vi "Manipulator Intake Handler.vi"(0 "Driver Axes":dbl[](array[numeric]), 1 "Driver Buttons":bool[](array[boolean]), 2 "Driver POVs":i16[](array[numeric]), 3 "Operator Axes":dbl[](array[numeric]), 4 "Operator Buttons":bool[](array[boolean]), 5 "Operator POVs":i16[](array[numeric])) -> ()   [LabVIEW 2020]
uses:
  <vilib>/Rock Robotics/WPI/Joystick/XBox Axes Indexer.ctl
  <vilib>/Rock Robotics/WPI/Joystick/XBox Buttons Indexer.ctl
  74f8955f-b1fa-4a71-b90e-be9672dc2c54.vi
  ec023221-8c5a-475e-8a5e-13ba12a89865.vi
  manipulator/Implementation/Typedefs/game object.ctl
  manipulator/Implementation/Typedefs/Cascade Height.ctl
  manipulator/Implementation/manipulator Operations.ctl
  manipulator/Implementation/Typedefs/Teleop Manipulator Commands.ctl
  52cbdbc3-376d-4ae6-b30b-ce1f15df8f80.vi
  dadffdc7-6345-417f-8810-915f08729db8.vi
  b64dc491-ae41-4b64-be03-725d494c7d40.vi
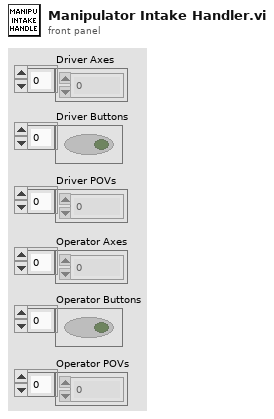
[diagram p1: front panel]
types:
  T1 = typedef "XBox Buttons Indexer.ctl" = enum16{"A", "B", "X", "Y", "Left Bumper", "Right Bumper", "Back", "Start", "Left Joystick", "Right Joystick"}
  T2 = typedef "Teleop Manipulator Commands.ctl" = enum16{"idle", "intake cone", "intake cube", "score low cone", "score low cube", "score mid cone", "score mid cube", "score high cone", "score high cube"}
  T3 = typedef "manipulator Operations.ctl" = enum16{"Reserve", "Read Current", "Immediate", "Reset Manipulator", "Grid-dy"}
  T4 = typedef "XBox Axes Indexer.ctl" = enum16{"Left X", "Left Y", "Left Trigger", "Right Trigger", "Right X", "Right Y"}
  T5 = typedef "game object.ctl" = enum16{"cone", "cube"}
  T6 = typedef "Cascade Height.ctl" = enum16{"Middle", "High"}
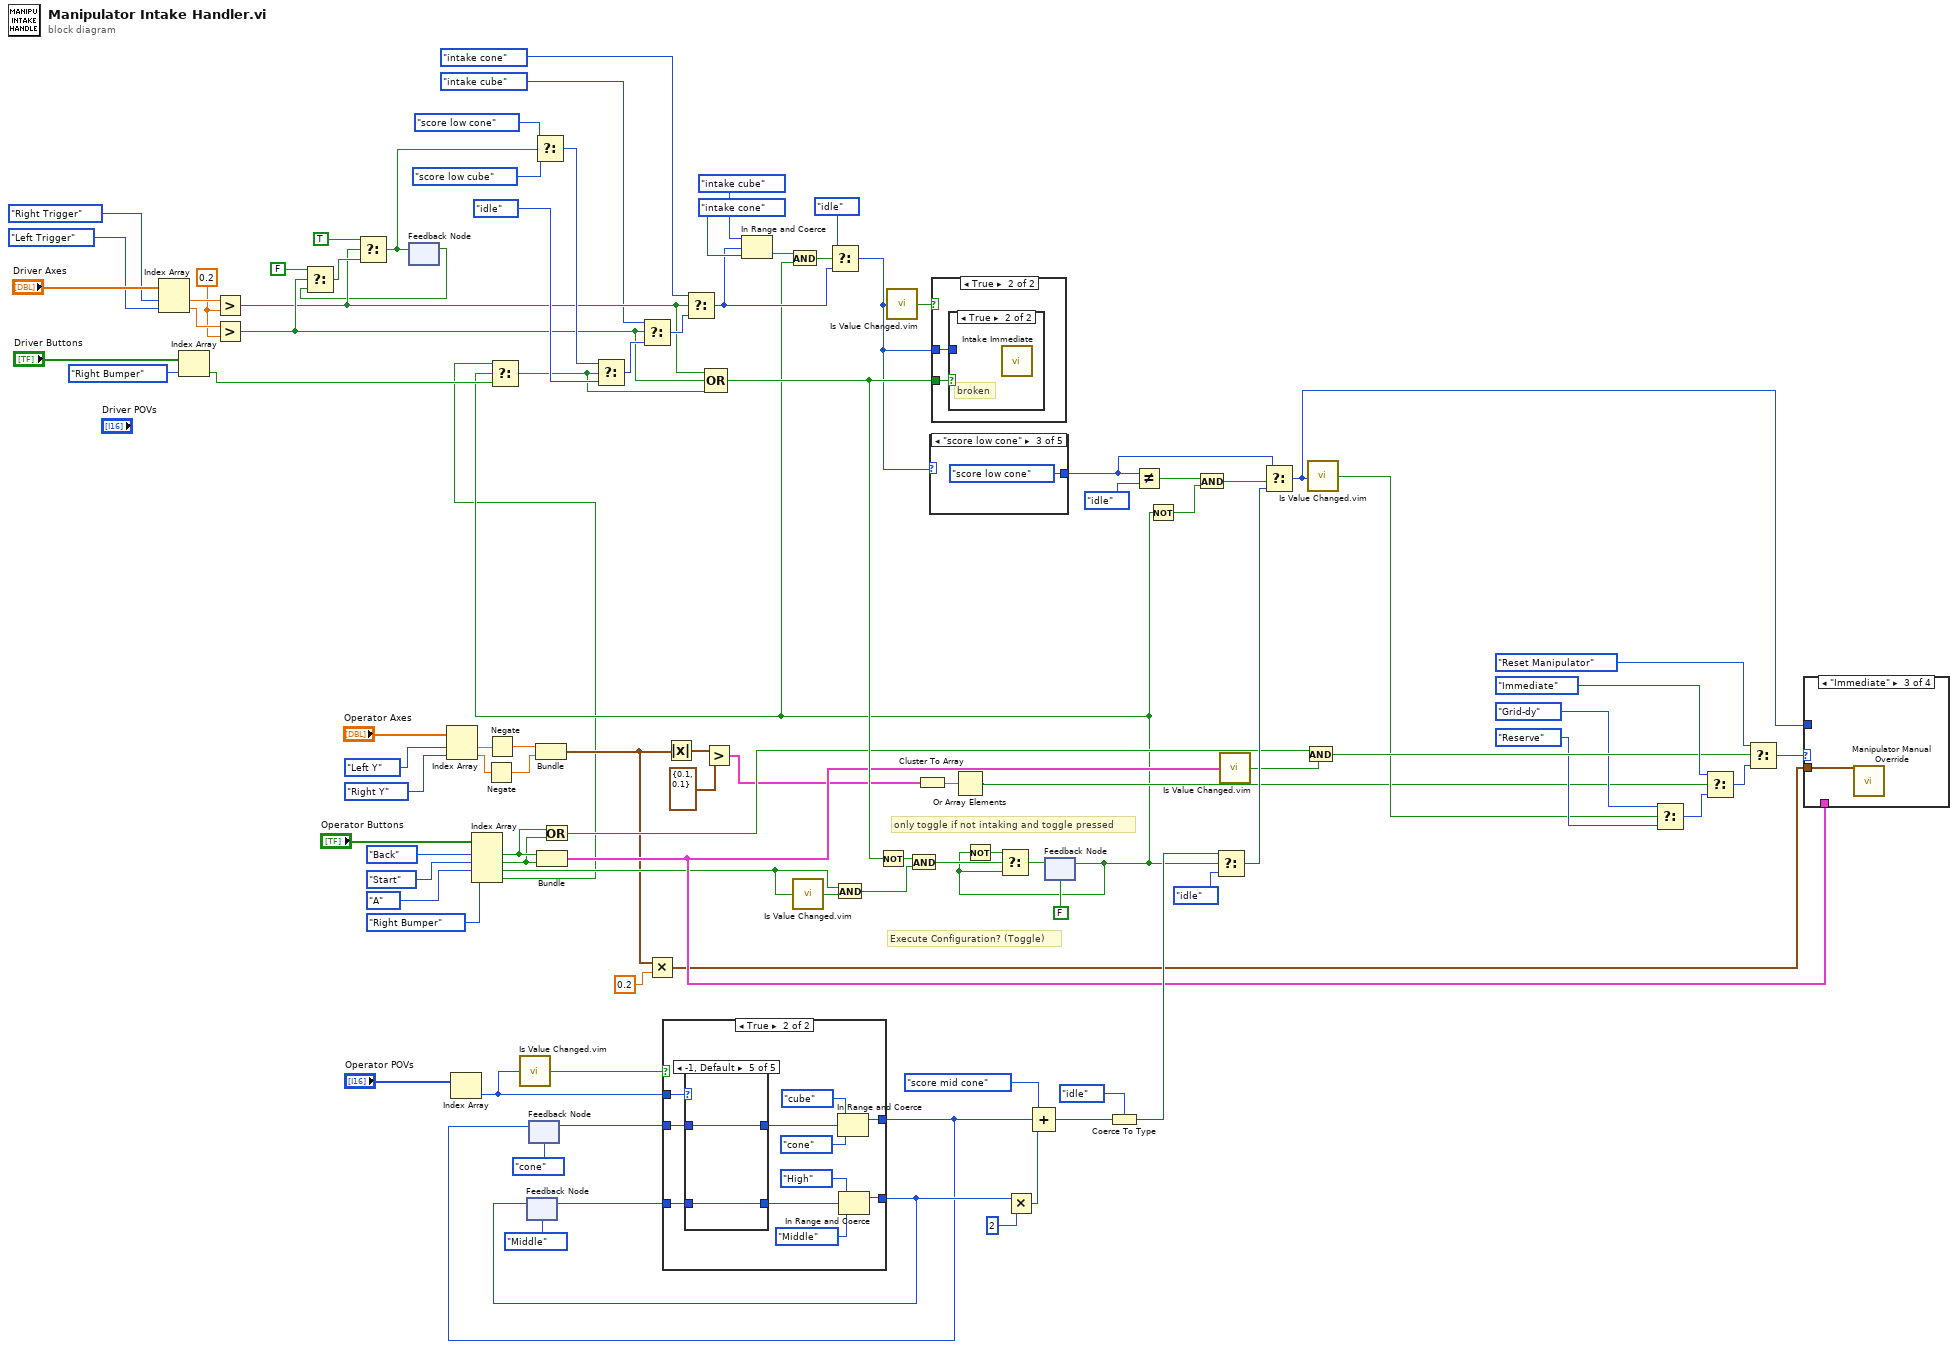
[diagram p0: block diagram]
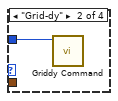
[diagram p3: hidden frame]
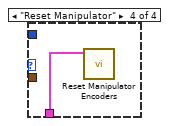
[diagram p4: hidden frame]
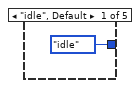
[diagram p5: hidden frame]
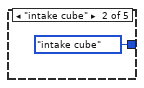
[diagram p6: hidden frame]
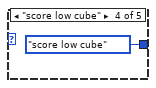
[diagram p7: hidden frame]
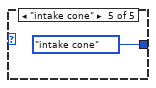
[diagram p8: hidden frame]
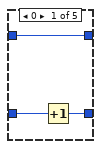
[diagram p10: hidden frame]
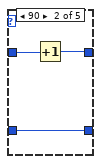
[diagram p11: hidden frame]
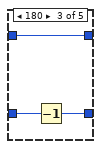
[diagram p12: hidden frame]
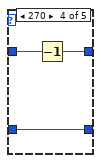
[diagram p13: hidden frame]
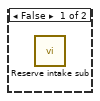
[diagram p15: hidden frame]
diagram:
  w96 = 0.2 ("y")
  # "only toggle if not intaking and toggle pressed"
  # "Execute Configuration? (Toggle)"
  n1 = Index Array(array="Driver Axes", index #1=XBox_Axes_Indexer."Right Trigger" ("XBox Axes"), index #2=XBox_Axes_Indexer."Left Trigger" ("XBox Axes")) -> (element #1=w98:dbl, element #2=w97:dbl)
  n2 = Index Array(array="Driver Buttons", index=XBox_Buttons_Indexer."Right Bumper" ("XBox Buttons")) -> (element=w4:bool)
  n3 = Greater?(x=w98, y=w96) -> (0:w31:bool)
  n4 = Greater?(x=w97, y=w96) -> (0:w33:bool)
  n5 = feedback #1() -> (w28:bool)  [unwired: 1 in]
  n6 = Select(t=FALSE, s=w33, f=w28) -> (s? t:f=w32:bool)
  n7 = Select(t=TRUE, s=w31, f=w32) -> (s? t:f=w27:bool)
  n8 = feedback-in #1(w27) -> ()
  n9 = Index Array(array="Operator Axes", index #1=XBox_Axes_Indexer."Left Y" ("XBox Axes"), index #2=XBox_Axes_Indexer."Right Y" ("XBox Axes")) -> (element #1=w80:dbl, element #2=w79:dbl)
  n10 = Index Array(array="Operator POVs") -> (element=w89:i16)  [unwired: 1 in]
  n11 = Index Array(array="Operator Buttons", index #1=XBox_Buttons_Indexer."Back" ("XBox Buttons"), index #2=XBox_Buttons_Indexer."Start" ("XBox Buttons"), index #3=XBox_Buttons_Indexer."A" ("XBox Buttons"), index #4=XBox_Buttons_Indexer."Right Bumper" ("XBox Buttons")) -> (element #1=w69:bool, element #2=w68:bool, element #3=w15:bool, element #4=w1:bool)
  n12 = Negate(x=w79) -> (-x=w74:dbl)
  n13 = Negate(x=w80) -> (-x=w75:dbl)
  n14 = call "Is Value Changed.vim"("value"=w89) -> ("changed or first call?"=w88:bool)
  n15 = feedback #2(Cascade_Height."Middle") -> (w85:T6)
  n16 = feedback #3(game_object."cone" ("Enum")) -> (w87:T5)
  n17 = Select(t=Teleop_Manipulator_Commands."score low cone" ("grid-dy commands"), s=w27, f=Teleop_Manipulator_Commands."score low cube" ("grid-dy commands")) -> (s? t:f=w36:T2)
  n18 = Bundle(w75, w74) -> (w14:cluster{dbl, dbl})  [unwired: 1 in]
  n19 = Bundle(w69, w68) -> (w37:cluster{bool, bool})  [unwired: 1 in]
  n20 = Or(x=w69, y=w68) -> (x .or. y?=w45:bool)
  n21 = Multiply(x=w14, y=0.2) -> (x*y=w13:cluster{dbl, dbl})
  n22 = case shown="True" w88 {
    tunnel: w89 -> [_ w114]
    tunnel: w87 -> [w103 w113]
    tunnel: w85 -> [w102 w112]
    tunnel: [w103 w110] -> w54
    tunnel: [w102 w106] -> w56
    frame False {
    }
    frame True {
      n23 = case shown="-1, Default" w114 {
        tunnel: w113 -> [w116 w119 w121 w126 w128]
        tunnel: w112 -> [w117 w120 w123 w124 w127]
        tunnel: [w115 w120 w122 w124 w127] -> w109
        tunnel: [w116 w118 w121 w125 w128] -> w111
        frame 0 {
          n24 = Increment(x=w117) -> (x+1=w115:T6)
        }
        frame 90 {
          n25 = Increment(x=w119) -> (x+1=w118:T5)
        }
        frame 180 {
          n26 = Decrement(x=w123) -> (x-1=w122:T6)
        }
        frame 270 {
          n27 = Decrement(x=w126) -> (x-1=w125:T5)
        }
        frame -1, Default {
        }
      }
      n28 = In Range and Coerce(upper limit=game_object."cube" ("Enum"), x=w111, lower limit=game_object."cone" ("Enum")) -> (coerced(x)=w110:T5)  [unwired: 1 out]
      n29 = In Range and Coerce(upper limit=Cascade_Height."High", x=w109, lower limit=Cascade_Height."Middle") -> (coerced(x)=w106:T6)  [unwired: 1 out]
    }
  }
  n30 = feedback-in #2(w56) -> ()
  n31 = feedback-in #3(w54) -> ()
  n32 = Absolute Value(x=w14) -> (abs(x)=w38:cluster{dbl, dbl})
  n33 = Greater?(x=w38, y=cluster{dbl, dbl} {0.1, 0.1}) -> (0:w9:cluster{bool, bool})
  n34 = call "Is Value Changed.vim"("value"=w15) -> ("changed or first call?"=w17:bool)
  n35 = And(x=w15, y=w17) -> (x .and. y?=w16:bool)
  n36 = Cluster To Array(cluster=w9) -> (array=w11:bool[])
  n37 = Or Array Elements(Boolean array=w11) -> (logical OR=w10:bool)
  n38 = Multiply(x=w56, y=2) -> (x*y=w52:i32)
  n39 = Compound Arithmetic op=ADD(Teleop_Manipulator_Commands."score mid cone" ("y"), w54, w52) -> (w50:i32)
  n40 = feedback #4(FALSE) -> (w2:bool)
  n41 = Select(t=w1, s=w2, f=w4) -> (s? t:f=w3:bool)
  n42 = Select(t=w36, s=w3, f=Teleop_Manipulator_Commands."idle" ("grid-dy commands")) -> (s? t:f=w92:T2)
  n43 = Select(t=Teleop_Manipulator_Commands."intake cube" ("grid-dy commands"), s=w33, f=w92) -> (s? t:f=w93:T2)
  n44 = Select(t=Teleop_Manipulator_Commands."intake cone" ("grid-dy commands"), s=w31, f=w93) -> (s? t:f=w19:T2)
  n45 = Compound Arithmetic op=OR(w31, w33, w3) -> (w61:bool)
  n46 = In Range and Coerce(upper limit=Teleop_Manipulator_Commands."intake cube", x=w19, lower limit=Teleop_Manipulator_Commands."intake cone") -> (In Range?=w21:bool)  [unwired: 1 out]
  n47 = And(x=w21, y=w2) -> (x .and. y?=w20:bool)
  n48 = Select(t=Teleop_Manipulator_Commands."idle", s=w20, f=w19) -> (s? t:f=w18:T2)
  n49 = Not(x=w61) -> (.not. x?=w63:bool)
  n50 = call "Is Value Changed.vim"("value"=w18) -> ("changed or first call?"=w91:bool)
  n51 = And(x=w63, y=w16) -> (x .and. y?=w62:bool)
  n52 = case shown="\"score low cone\"" w18 {
    tunnel: [Teleop_Manipulator_Commands."idle" ("grid-dy commands") Teleop_Manipulator_Commands."intake cube" ("grid-dy commands") Teleop_Manipulator_Commands."score low cone" ("grid-dy commands") Teleop_Manipulator_Commands."score low cube" ("grid-dy commands") Teleop_Manipulator_Commands."intake cone" ("grid-dy commands")] -> w58
    frame "idle", Default {
    }
    frame "intake cube" {
    }
    frame "score low cone" {
    }
    frame "score low cube" {
    }
    frame "intake cone" {
    }
  }
  n53 = case shown="True" w91 {
    tunnel: w18 -> [_ w134]
    tunnel: w61 -> [_ w135]
    frame False {
    }
    frame True {
      n54 = case shown="True" w135 {
        tunnel: w134 -> [_ _]
        frame False {
          n55 = call "Reserve intake sub.vi"() -> ()  [unwired: 11 in, 1 out]
        }
        frame True {
          # "broken"
          n56 = call "Intake Immediate.vi"() -> ()  [unwired: 11 in, 1 out]
        }
      }
    }
  }
  n57 = Not(x=w2) -> (.not. x?=w66:bool)
  n58 = Select(t=w66, s=w62, f=w2) -> (s? t:f=w65:bool)
  n59 = feedback-in #4(w65) -> ()
  n60 = Coerce To Type(0:w50, 1:Teleop_Manipulator_Commands."idle" ("y")) -> (2:w49:T2)
  n61 = Not Equal?(x=w58, y=Teleop_Manipulator_Commands."idle") -> (x != y?=w8:bool)
  n62 = Not(x=w2) -> (.not. x?=w7:bool)
  n63 = And(x=w8, y=w7) -> (x .and. y?=w6:bool)
  n64 = Select(t=w49, s=w2, f=Teleop_Manipulator_Commands."idle") -> (s? t:f=w57:T2)
  n65 = call "Is Value Changed.vim"("value"=w37) -> ("changed or first call?"=w46:bool)
  n66 = Select(t=w58, s=w6, f=w57) -> (s? t:f=w39:T2)
  n67 = And(x=w45, y=w46) -> (x .and. y?=w47:bool)
  n68 = call "Is Value Changed.vim"("value"=w39) -> ("changed or first call?"=w41:bool)
  n69 = Select(t=manipulator_Operations."Grid-dy" ("Operation"), s=w41, f=manipulator_Operations."Reserve" ("Operation")) -> (s? t:f=w42:T3)
  n70 = Select(t=manipulator_Operations."Immediate" ("Operation"), s=w10, f=w42) -> (s? t:f=w70:T3)
  n71 = Select(t=manipulator_Operations."Reset Manipulator" ("Operation"), s=w47, f=w70) -> (s? t:f=w40:T3)
  n72 = case shown="\"Immediate\"" w40 {
    tunnel: w37 -> [_ _ _ w138]
    tunnel: w39 -> [_ w136 _ _]
    tunnel: w13 -> [_ _ w137 _]
    frame "Reserve", Default {
    }
    frame "Grid-dy" {
      n73 = call "Griddy Command.vi"("Griddy Command"=w136) -> ()  [unwired: 10 in, 1 out]
    }
    frame "Immediate" {
      n74 = call "Manipulator Manual Override.vi"("Immediate Parameters"=w137) -> ()  [unwired: 10 in, 1 out]
    }
    frame "Reset Manipulator" {
      n75 = call "Reset Manipulator Encoders.vi"("Reset Parameters"=w138) -> ()  [unwired: 10 in, 1 out]
    }
  }
